vi "test_Multiple Static Response Messages using Trigger and Wait Byte Count from a Channel.vi"(8 "error in (no error)":errorcluster, 11 "TestCase in":refnum<class "Instrument Addon Common System Tests.lvclass">) -> (0 "error out":errorcluster, 3 "TestCase out":refnum<class "Instrument Addon Common System Tests.lvclass">)   [LabVIEW 2019, in "Instrument Addon Common System Tests.lvclass"]
uses:
  Instrument Addon Common System Tests.lvclass
  <vilib>/addons/_JKI Toolkits/VI Tester/TestCase.llb/TestCase.lvclass
  <vilib>/NI VeriStand/Execution/Workspace/NI_VS Workspace ExecutionAPI.lvlib
  <vilib>/NI VeriStand/Execution/Workspace/NI VeriStand - Get Multiple Channel Values.vi
  <vilib>/NI VeriStand/Execution/Workspace/NI VeriStand - Set Multiple Channel Values.vi
  C:/Users/nitest/Desktop/Git 2019/niveristand-custom-device-testing-tools/VeriStandTestCase/VeriStandTestCase.lvclass
  C:/Program Files (x86)/National Instruments/LabVIEW 2019/vi.lib/addons/_JKI Toolkits/VI Tester/TestCase.llb/TestCase.lvclass
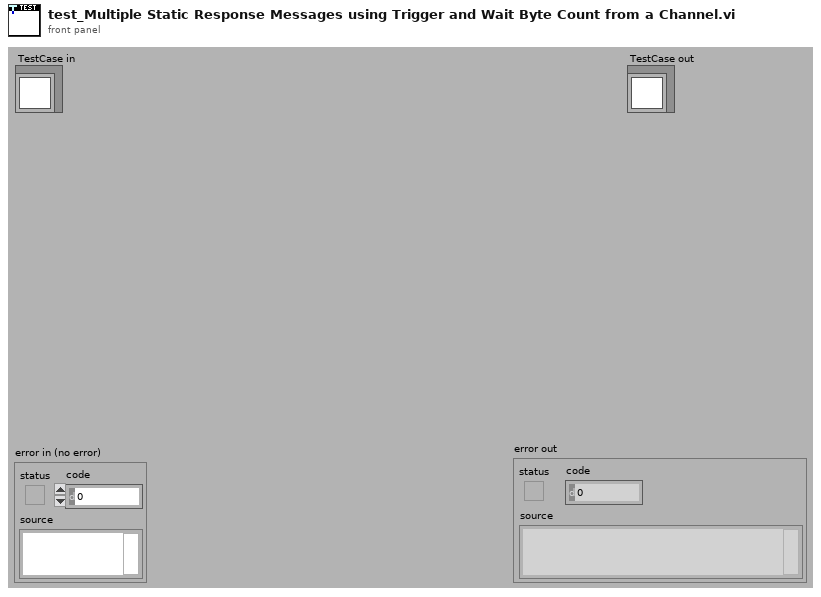
[diagram p1: front panel]
types:
  T1 = typedef "NI_VS Workspace ExecutionAPI.lvlib/WorkspaceAPI.ctl" = refnum<k24>
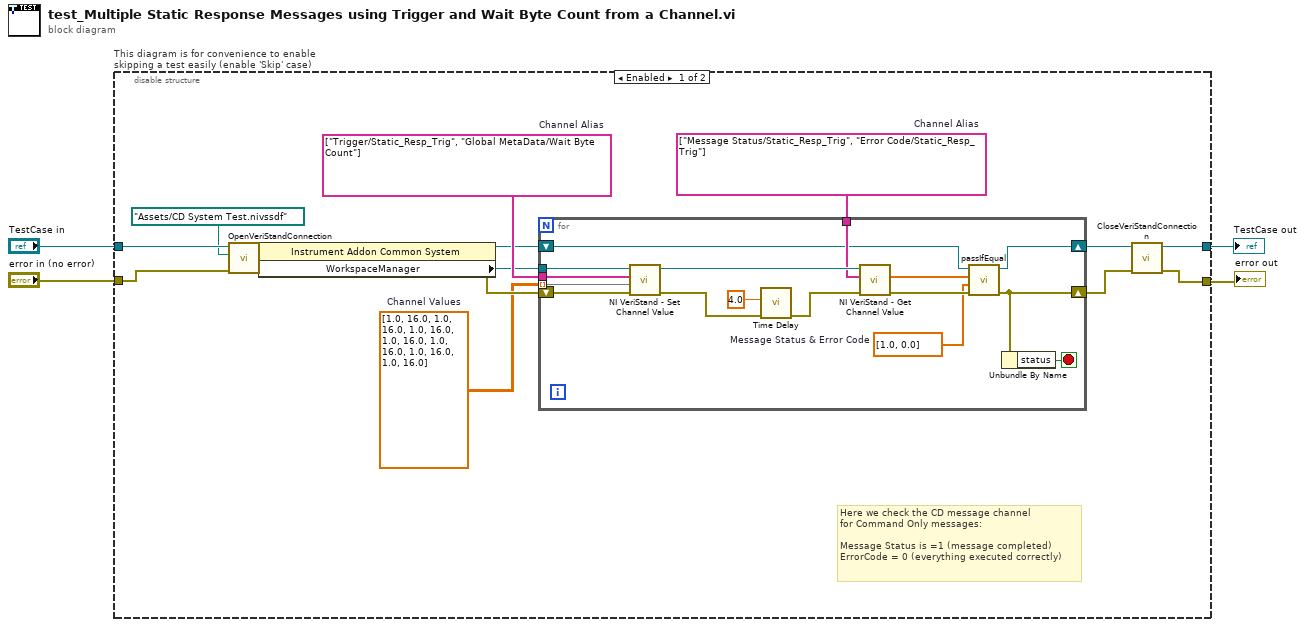
[diagram p0: block diagram]
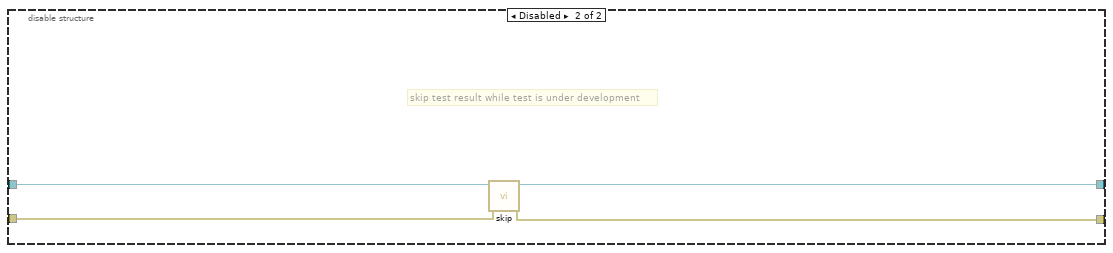
[diagram p2: hidden frame]
diagram:
  n1 = disable-structure "This diagram is for convenience to enable skipping a test easily (enable 'Skip' case)" shown="Enabled" {
    disable-tunnel: "TestCase in" -> [w17 w39]
    disable-tunnel: [w18 w37] -> w1
    disable-tunnel: [w19 w38] -> w3
    disable-tunnel: "error in (no error)" -> [w15 w36]
    frame Enabled {
      w8 = string[] ["Message Status/Static_Resp_Trig", "Error Code/Static_Resp_Trig"]  # Channel Alias
      w10 = dbl[][] [[1.0, 16.0], [1.0, 16.0], [1.0, 16.0], [1.0, 16.0], [1.0, 16.0], [1.0, 16.0], [1.0, 16.0]]  # Channel Values
      w11 = string[] ["Trigger/Static_Resp_Trig", "Global MetaData/Wait Byte Count"]  # Channel Alias
      # "Here we check the CD message channel\nfor Command Only messages:\n\nMessage Status is =1 (message completed)\nErrorCode = 0 (everything executed correctly)"
      n2 = call-dynamic "OpenVeriStandConnection.vi"("error in (no error)"=w15, "System Definition File"=path "Assets/CD System Test.nivssdf", "VeriStand Test Case in"=w17) -> ("error out"=w14:errorcluster, "VeriStand Test Case out"=w16:refnum<class "Instrument Addon Common System Tests.lvclass">)  [unwired: 6 in, 1 out]
      n3 = property class="Instrument Addon Common System "(reference=w16, error in=w14) -> (reference out=w9:refnum<class "Instrument Addon Common System Tests.lvclass">, error out=w12:errorcluster, "WorkspaceManager"=w7:T1)
      n4 = for {
        tunnel: w7 -> [w35]
        tunnel: w11 -> [w33]
        tunnel: w10 -> [w21] mode=indexing
        shift-right: [w20] -> w5
        shift-left: w12 -> [w34]
        tunnel: w8 -> [w31]
        shift-right: [w26] -> w6
        shift-left: w9 -> [w27]
        stop <- w23 stop-if-true
        w22 = dbl[] [1.0, 0.0]  # Message Status & Error Code
        n5 = call-poly <vilib>:"NI VeriStand - Set Channel Value.vi"("error in (no error)"=w34, "Values"=w21, "Channels"=w33, "WorkspaceManager in"=w35) -> ("error out"=w29:errorcluster, "WorkspaceManager out"=w32:T1)  [unwired: 6 in]
        n6 = call "Time Delay"("error in (no error)"=w29, "Delay Time (s)"=4.0) -> ("error out"=w28:errorcluster)  [unwired: 9 in]
        n7 = call-poly <vilib>:"NI VeriStand - Get Channel Value.vi"("error in (no error)"=w28, "Channels"=w31, "WorkspaceManager in"=w32) -> ("error out"=w25:errorcluster, "Values"=w24:dbl[])  [unwired: 6 in, 1 out]
        n8 = call-dynamic "passIfEqual.vi"("error in (no error)"=w25, "y"=w22, "x"=w24, "TestCase in"=w27) -> ("error out"=w20:errorcluster, "TestCase out"=w26:refnum<class "Instrument Addon Common System Tests.lvclass">)  [unwired: 6 in]
        n9 = Unbundle By Name(w20) -> ("status"=w23:bool)
      }
      n10 = call-dynamic "CloseVeriStandConnection.vi"("error in (no error)"=w5, "VeriStand Test Case in"=w6) -> ("error out"=w19:errorcluster, "VeriStand Test Case out"=w18:refnum<class "Instrument Addon Common System Tests.lvclass">)  [unwired: 8 in]
    }
    frame Disabled {
      # "skip test result while test is under development"
      n11 = call <vilib>:"skip.vi"("error in (no error)"=w36, "TestCase in"=w39) -> ("error out"=w38:errorcluster, "TestCase out"=w37:refnum<class "Instrument Addon Common System Tests.lvclass">)  [unwired: 8 in]
    }
  }
  "error out" <- w3
  "TestCase out" <- w1
